vi "Receive.vi"(7 "Actor in":refnum<class "Actor.lvclass">, 9 "From Msg Event":bool, 10 "Msg":refnum<class "Msg.lvclass">) -> (0 "Error out":errorcluster, 5 "Actor out":refnum<class "Actor.lvclass">)   [LabVIEW 2025, in "jettl.lvlib" / "Actor.lvlib"]
uses:
  Actor.lvlib
  Actor/Actor.lvclass
  Msg/Msg.lvclass
  Attributes/Attributes/Attributes.lvclass
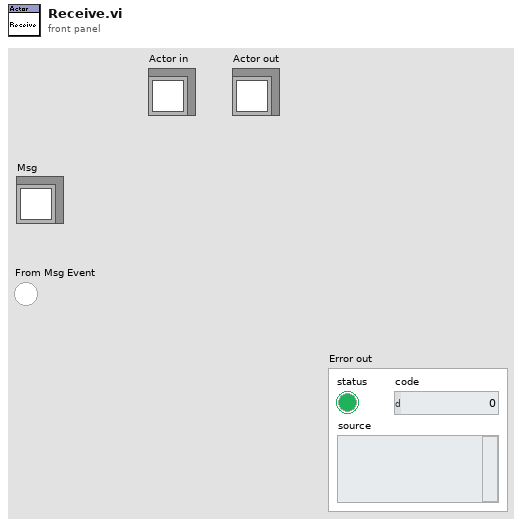
[diagram p1: front panel]
types:
  T1 = typedef "jettl.lvlib/Actor.lvlib/Msg Set.ctl" = set{refnum<class "Msg.lvclass">}
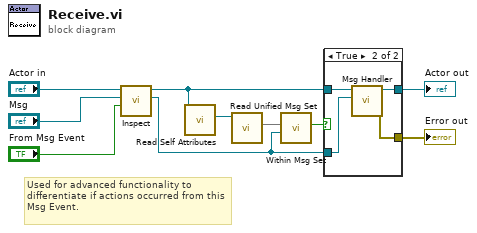
[diagram p0: block diagram]
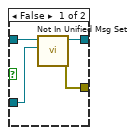
[diagram p2: hidden frame]
diagram:
  # "Used for advanced functionality to differentiate if actions occurred from this Msg Event."
  n1 = call-dynamic "Inspect.vi"("From Msg Event"="From Msg Event", "Msg in"="Msg", "Actor in"="Actor in") -> ("Msg out"=w2:refnum<class "Msg.lvclass">, "Actor out"=w4:refnum<class "Actor.lvclass">)  [unwired: 7 in]
  n2 = call-dynamic "Read Self Attributes.vi"("Actor in"=w4) -> ("Self Attributes"=w10:refnum<class "Attributes.lvclass">)  [unwired: 10 in]
  n3 = call-dynamic "Read Unified Msg Set.vi"("Attributes in"=w10) -> ("Unified Msg Set"=w9:T1)  [unwired: 10 in]
  n4 = call "Within Msg Set.vi"("Msg"=w2, "Msg Set"=w9) -> ("Within Msg Set"=w8:bool)  [unwired: 9 in]
  n5 = case shown="True" w8 {
    tunnel: w4 -> [w14 w18]
    tunnel: [w13 w16] -> w7
    tunnel: w2 -> [w11 w17]
    tunnel: [w12 w15] -> w6
    frame False {
      n6 = call-dynamic "Not In Unified Msg Set.vi"("Msg"=w11, "Actor in"=w14) -> ("Error out"=w12:errorcluster, "Actor out"=w13:refnum<class "Actor.lvclass">)  [unwired: 8 in]
    }
    frame True {
      n7 = call-dynamic "Msg Handler.vi"("Msg"=w17, "Actor in"=w18) -> ("Error out"=w15:errorcluster, "Actor out"=w16:refnum<class "Actor.lvclass">)  [unwired: 8 in]
    }
  }
  "Actor out" <- w7
  "Error out" <- w6
